vi "BITalino.vi"() -> ()   [LabVIEW 2019]
uses:
  Status.ctl
  Sensor.ctl
  <vilib>/Instr/_visa.llb/VISA Configure Serial Port (Instr).vi
  <vilib>/measure/mamon.llb/Waveform Peak Detection for N Chan.vi
  <vilib>/httpClient/LabVIEWHTTPClient.lvlib
  <vilib>/measure/NI_MAPro.lvlib
panel:
  in  "Tab Control":T1(tab)
  in  "Entrer":bool
  in  "fermer":bool
  in  "reset":bool
  in  "Login":bool
  in  "Pass Word":string
  in  "User Name":string
  in  "Search Button 2":bool
  in  "acquisition 2":bool
  in  "fermer 3":bool
  in  "Home Button":bool
  in  "inscription":bool
  in  "acquisition":bool
  in  "documentation":bool
  in  "Refresh Button2":bool
  in  "Open Button":bool
  in  "Search Button":bool
  in  "fermer 4":bool
  in  "suivant":bool
  in  "sexe":string
  in  "Age":string
  in  "nom":string
  in  "CIN":string
  in  "prenom":string
  in  "Refresh":bool
  in  "envoyer":bool
  out "body":string
  in  "Home Button 2":bool
  out "body 2":string
  in  "CIN":string
  out "body 3":string
  in  "Previous Button":bool
  in  "Jump Button":bool
  in  "Stop Button":bool
  in  "Record Button":bool
  in  "Exit Button":bool
  out "Status":T2
  in  "Device":refnum<visa-resource-name>
  in  "X Limit":u32(knob)=5 scale=2.0..30.0
  in  "File Path":path
  in  "Sample Rate":enum16{"1", "10", "100", "1000"}(ring)=enum."1000"
  in  "MODE":bool
  out "DI 3":bool
  out "DI 4":bool
  out "DI 1":bool
  out "DI 2":bool
  in  "Sensor 1":T3
  in  "Sensor 2":T3=enum."ECG"
  in  "Sensor 3":T3=enum."EEG"
  in  "Sensor 4":T3=enum."EDA"
  in  "Sensor 5":T3=enum."ACC"
  in  "Sensor 6":T3=enum."LUX"
  in  "Sensor Selection":enum32{"A1", "A2", "A3", "A4", "A5", "A6"}(radio)
  out "XY Graph":cluster{dbl[], dbl[]}(graph)
  out "CRC Error":bool
  in  "Battery \nThreshold (%)":u8(slide)=5 min=5 max=90 step=5 scale=5.0..90.0
  in  "DO 1":bool
  in  "DO 2":bool
  in  "DO 3":bool
  in  "DO 4":bool
  in  "Home Button 3":bool
  out "ECG":string[][](table) caption="Table"
  in  "Previous Button 2":bool
  in  "Save Button":bool
  in  "Record Button 2":bool
  out "ecg normal":dbl[](graph)
  in  "Menu Ring":u16(ring) items=["normal", "p interval", "qrs interval", "p-r interval"]
  in  "Home Button 4":bool
  in  "fermer 2":bool
  out "Impulsion":dbl
  out "fréquence en Hz":dbl
  out "Battement de coeur (batt/min)":dbl
  in  "use system alert? (T)":bool=TRUE
  out "Waveform Graph":dynamicdata(graph)
  out "body 4":string
  in  "Jump Button 2":bool
  in  "Previous Button 3":bool
  in  "Home Button 5":bool
  in  "fermer 5":bool
  out "tdms file":refnum<k34>
  out "Ylabel and Plot name":cluster{string, string}
  out "Sample Rate Numeric":i32
  out "Consumer":i32
  out "producer":i32
  in  "error in (no error)":errorcluster
  out "Sync Stop":bool=TRUE
  # "Bienvenue"
  # "Authentification"
  # "Traitement de Signal ECG"
  # "Chercher un Patient"
  # "Formulaire d'inscription"
  # "nom:"
  # "prenom:"
  # "CIN:"
  # "Age:"
  # "Sexe:"
  # "Acquisition de Signal ECG"
  # "LIVE MODE"
  # "SIMULATED MODE"
  # "Hz"
  # "Signal ECG"
  # "Signal ECG"
  # "L'Électrocardiogramme (ECG) est un enregistrement de l'activité électrique du cœur"
  # "Le tracé électrique comporte des ondes et des intervalles entre les ondes :\n\nOnde P : elle correspond à la dépolarisation (et la contraction) des oreillettes. Sa durée (entre 0.08 et 0.1 s) \n\nIntervalle PR (ou PQ) : c'est le temps entre le début de P et le début du \" QRS \". Il est témoins du temps nécessaire à la transmission de l'influx électrique des oreillettes aux ventricules et qui dure 0.12 à 0.20 s.\n\nOnde QRS (appelée aussi complexe QRS) : elle correspond à la dépolarisation (la contraction) des ventricules. une durée de 0.06 à 0.1s.\n\nOnde T : elle correspond à l'essentiel de repolarisation (relaxation des ventricules) et commence juste après QRS et dure de 0.2 à 0.25 s.\n\nIntervalle QT : il est mesuré du débit de QRS à la fin du l'onde T et il correspond à l'ensemble de la repolarisation cardiaque."
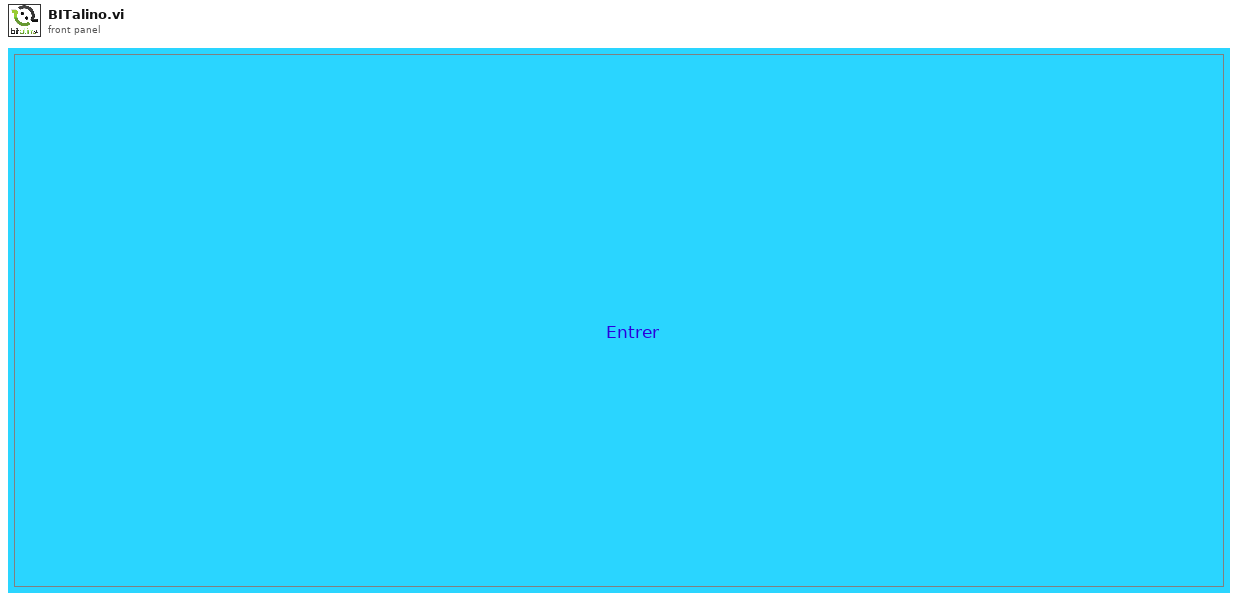
[diagram p1: front panel]
types:
  T1 = enum32{"bienvenue", "Authentification", "acueil", "inscription", "Acquisition", "simulation", "Documentation "}
  T2 = typedef "Status.ctl" = enum16{"Initialize", "Standby", "Recording", "Exit"}
  T3 = typedef "Sensor.ctl" = enum16{"EMG", "ECG", "EEG", "EDA", "ACC", "LUX"}
  T4 = enum8{"Enabled", "Disabled", "Disabled and Grayed Out"}
  T5 = enum16{"open", "open or create", "create or replace", "create", "open (read-only)"}
  T6 = cluster{"Sensor 1":T3, "Sensor 2":T3, "Sensor 3":T3, "Sensor 4":T3, "Sensor 5":T3, "Sensor 6":T3}
  T7 = cluster{"Result":dbl, "Result":dbl, "Result":dbl, "Result":dbl, "Result":dbl, "Result":dbl}
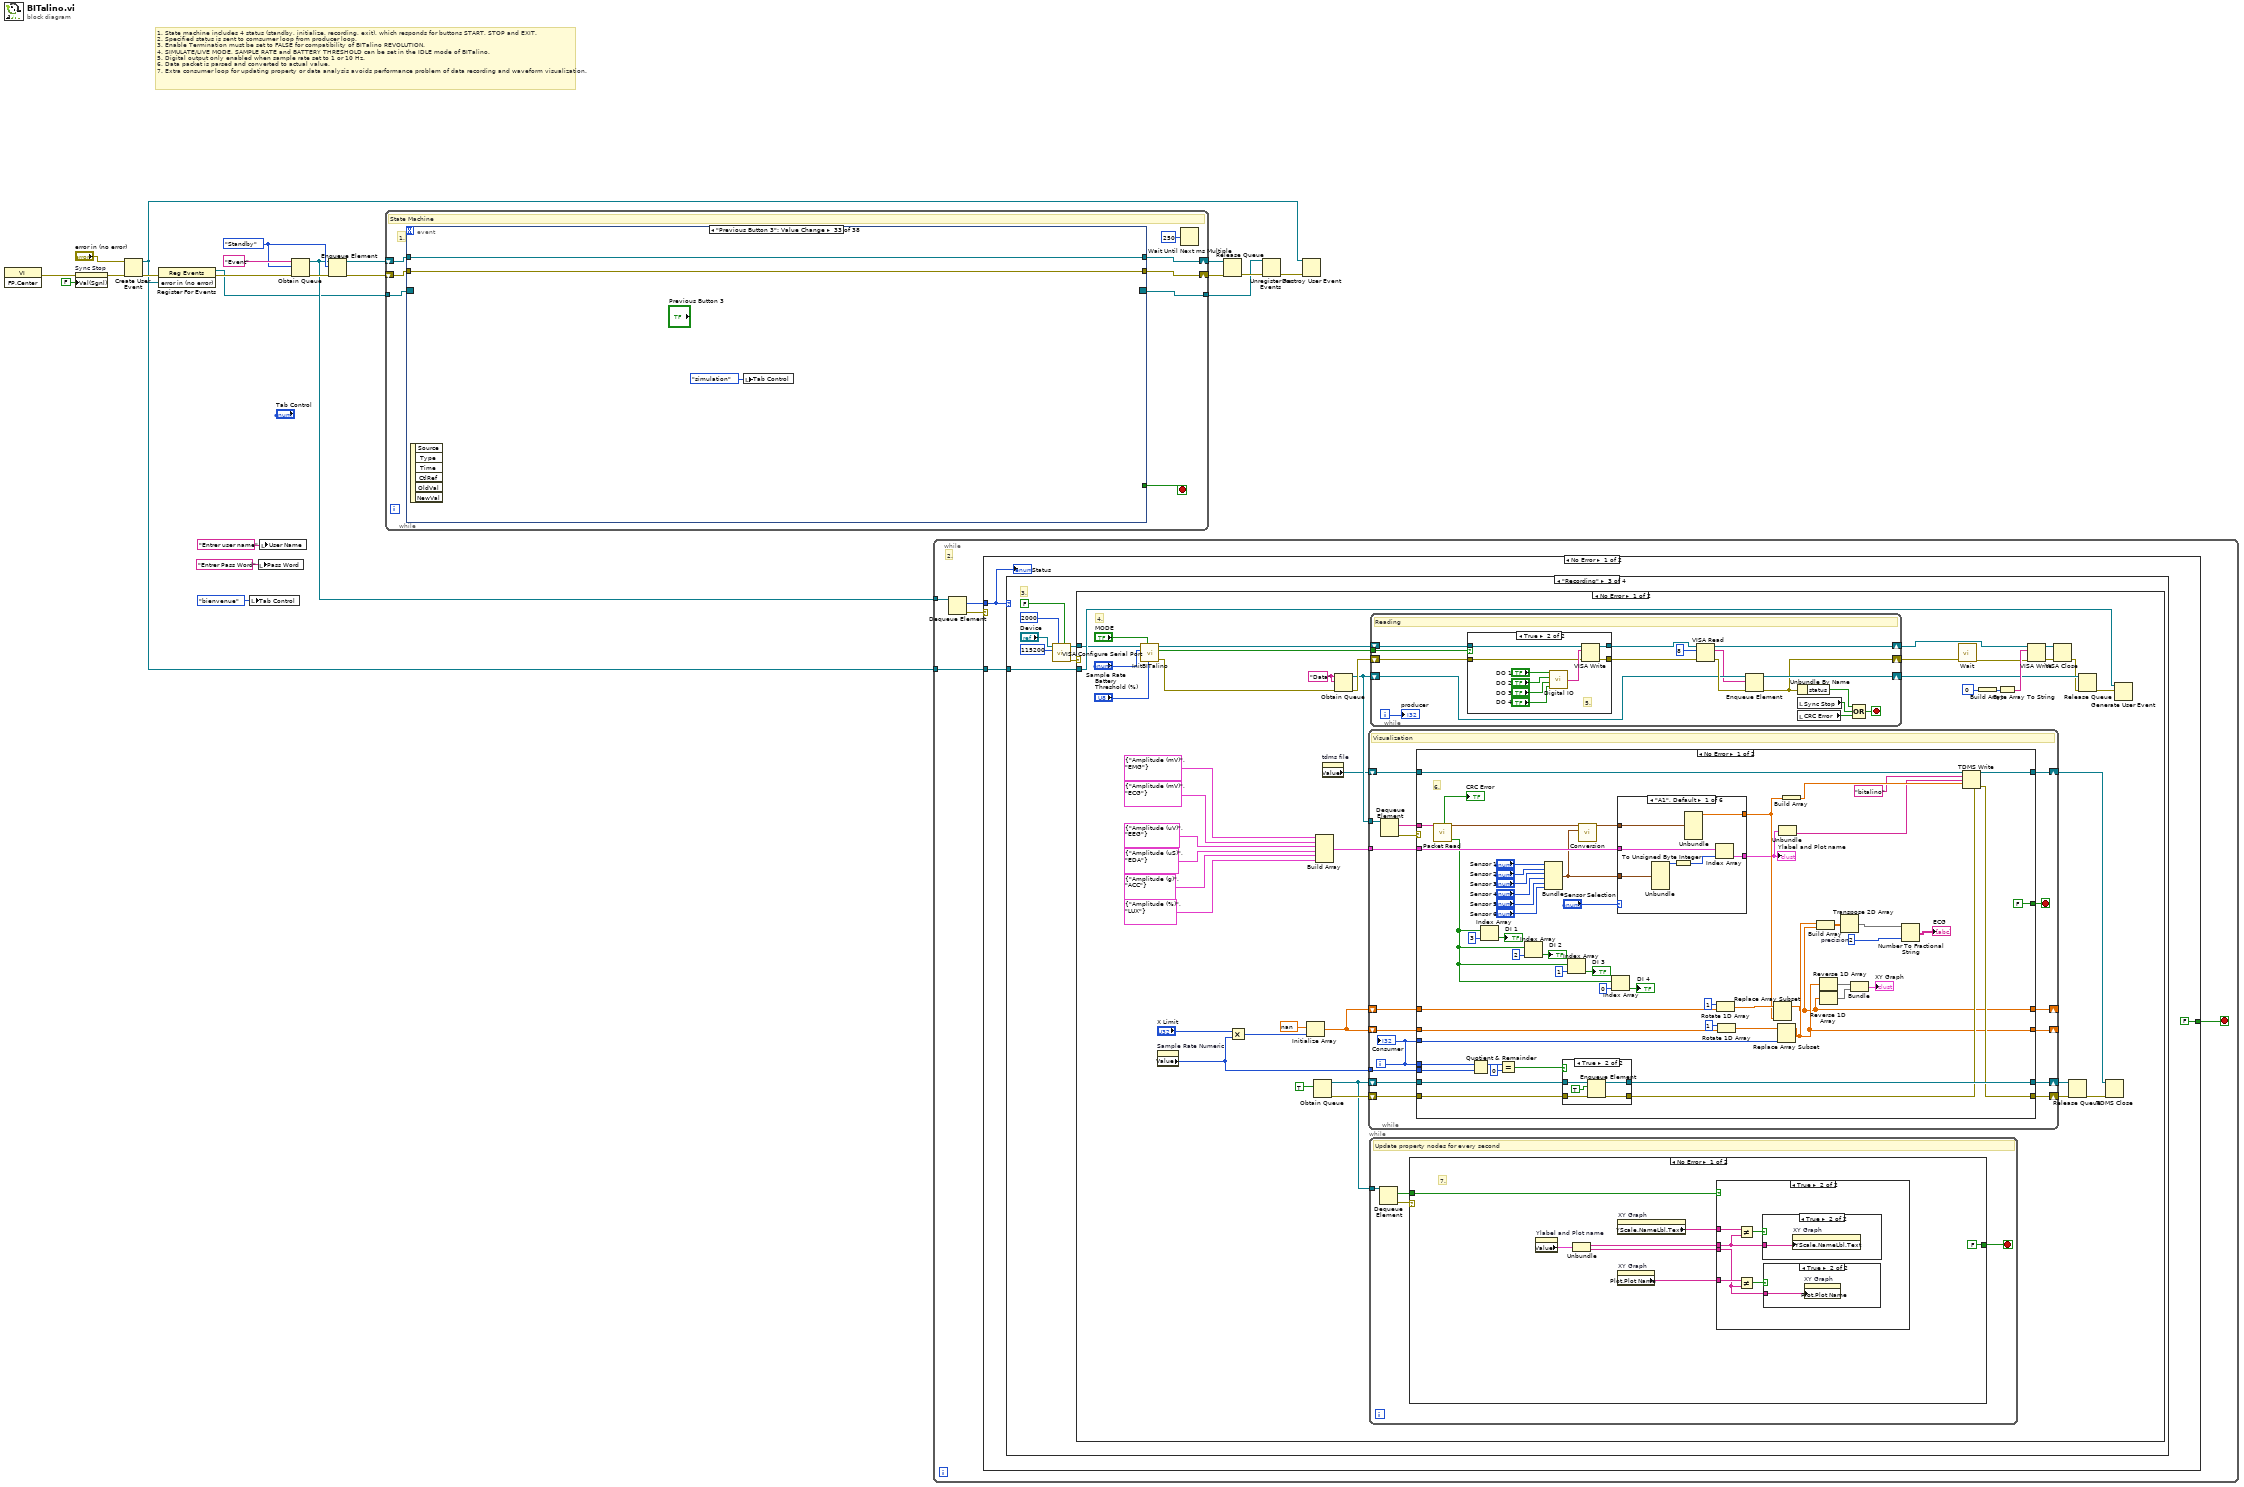
[diagram p0: block diagram]
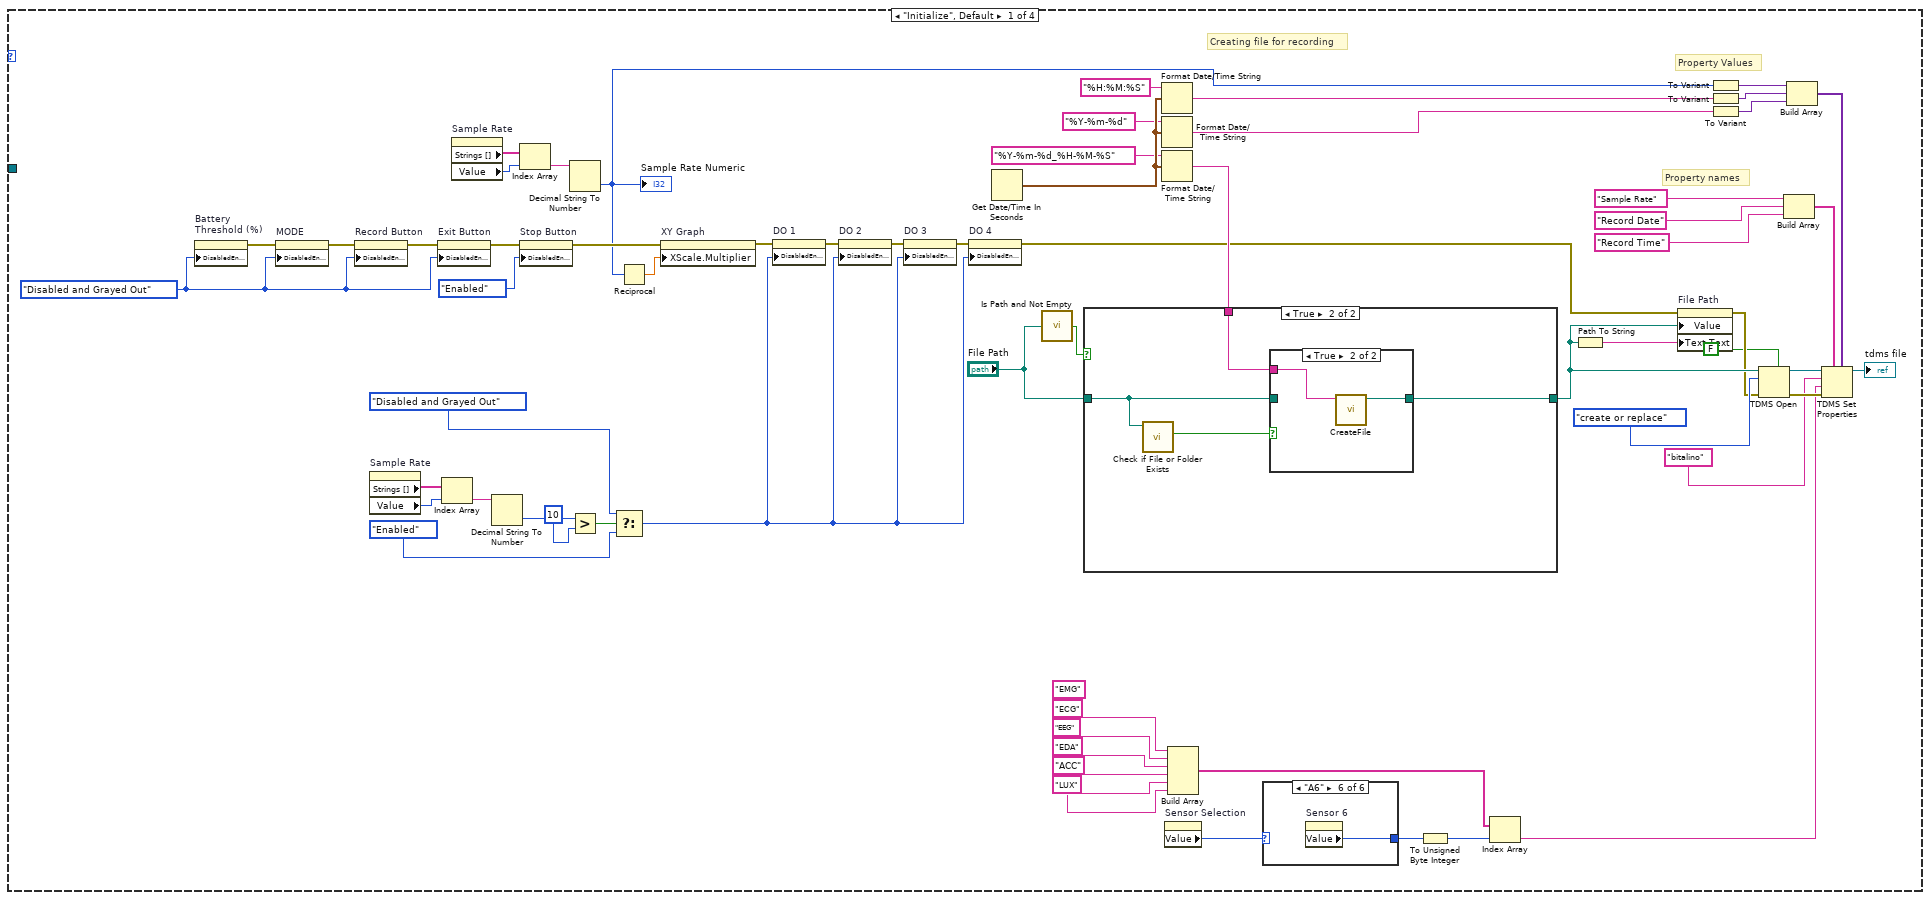
[diagram p2: hidden frame]
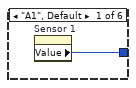
[diagram p3: hidden frame]
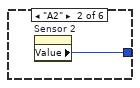
[diagram p4: hidden frame]
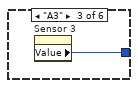
[diagram p5: hidden frame]
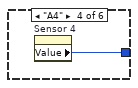
[diagram p6: hidden frame]
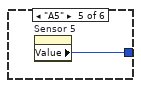
[diagram p7: hidden frame]
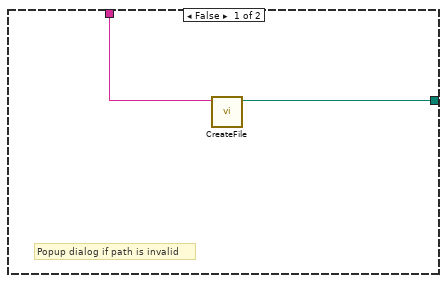
[diagram p8: hidden frame]
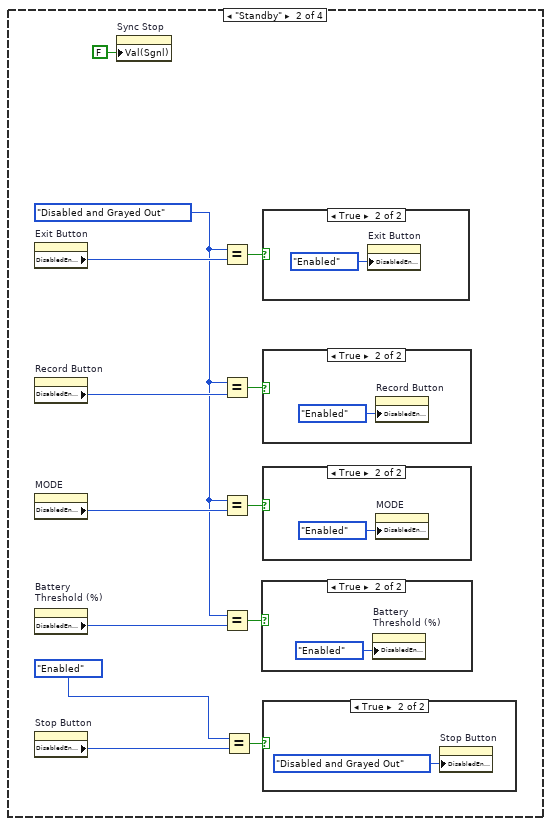
[diagram p10: hidden frame]
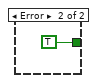
[diagram p19: hidden frame]
diagram:
  w16 = Status."Standby" ("Enum")
  # "1. State machine includes 4 status (standby, initialize, recording, exit), which responds for buttons START, STOP and EXIT.\n2. Specified status is sent to comsumer loop from producer loop.\n3. Enable Termination must be set to FALSE for compatibility of BITalino REVOLUTION.\n4. SIMULATE/LIVE MODE, SAMPLE RATE and BATTERY THRESHOLD can be set in the IDLE mode of BITalino.\n5. Digital output only enabled when sample rate set to 1 or 10 Hz.\n6. Data packet is parsed and converted to actual value.\n7. Extra consumer loop for updating property or data analysis avoids performance problem of data recording and waveform visualization."
  n1 = invoke class="VI" method="FP.Center"() -> (error out=w4:errorcluster)  [unwired: 3 in, 2 out]
  n2 = property on="Sync Stop" class="Bool (strict)"(error in=w4, "Val(Sgnl)"=FALSE ("Value (Signaling)")) -> (error out=w13:errorcluster)  [unwired: 1 in, 1 out]
  n3 = Create User Event(user event datatype="error in (no error)", error in=w13) -> (user event=w5:refnum<user-event>, error out=w12:errorcluster)
  n4 = register-events(error in=w12, w5) -> (reference out=w10:refnum<event-registration>, error out=w11:errorcluster)  [unwired: 1 in]
  n5 = local write "Tab Control"(T1."bienvenue" ("Tab Control")) -> ()
  n6 = local write "Pass Word"("Entrer Pass Word" ("Pass Word")) -> ()
  n7 = local write "User Name"("Entrer user name" ("User Name")) -> ()
  n8 = Obtain Queue(name (unnamed)="Event", element data type=w16, error in (no error)=w11) -> (queue out=w15:refnum<queue>, error out=w19:errorcluster)  [unwired: 2 in, 1 out]
  n9 = Enqueue Element(queue=w15, element=w16, error in (no error)=w19) -> (queue out=w17:refnum<queue>, error out=w18:errorcluster)  [unwired: 1 in, 1 out]
  n10 = while {
    shift-right: [w27] -> w21
    shift-left: w17 -> [w30]
    shift-right: [w28] -> w20
    shift-left: w18 -> [w29]
    tunnel: w10 -> [w24]
    tunnel: [w23] -> w7
    stop <- w26 stop-if-true
    # "1."
    # "State Machine"
    n11 = event shown="[32] \"Previous Button 3\": Value Change" {
      selector: w24 -> [_ _ _ _ _ _ _ _ _ _ _ _ _ _ _ _ _ _ _ _ _ _ _ _ _ _ _ _ _ _ _ _ _ _ _ _ _ _]
      dyn-events: [_ _ _ _ _ _ _ _ _ _ _ _ _ _ _ _ _ _ _ _ _ _ _ _ _ _ _ _ _ _ _ _ _ _ _ _ _ _] -> w23
      timeout: _ -> [_ _ _ _ _ _ _ _ _ _ _ _ _ _ _ _ _ _ _ _ _ _ _ _ _ _ _ _ _ _ _ _ _ _ _ _ _ _]
      tunnel: w30 -> [w37 w40 w57 w60 w63 w66 w69 w72 w75 w78 w84 w86 w89 w92 w104 w107 w109 w113 w128 w135 w144 w147 w172 w186 w194 w197 w200 w203 w206 w210 w213 w216 w219 w223 w227 w231 w241 w245]
      tunnel: w29 -> [w34 w39 w56 w59 w62 w65 w68 w71 w74 w80 w83 w85 w88 w91 w103 w106 w108 w112 w129 w136 w145 w148 w173 w185 w193 w198 w201 w204 w207 w211 w214 w217 w220 w224 w228 w232 w240 w243]
      tunnel: [w31 w39 w56 w59 w62 w65 w68 w71 w74 w81 w83 w85 w88 w91 w103 w106 w108 w112 w129 w136 w145 w148 w173 w185 w193 w198 w201 w204 w207 w211 w214 w217 w220 w224 w228 w232 w235 w242] -> w28
      tunnel: [w38 w40 w57 w60 w63 w66 w69 w72 w75 w79 w84 w86 w89 w92 w104 w107 w109 w113 w128 w135 w144 w147 w172 w186 w194 w197 w200 w203 w206 w210 w213 w216 w219 w223 w227 w231 w237 w244] -> w27
      tunnel: [FALSE _ _ _ _ _ _ _ _ TRUE _ _ _ _ _ _ _ _ _ _ _ _ _ _ _ TRUE _ _ _ TRUE _ _ _ TRUE TRUE TRUE FALSE _] -> w26
      event "Stop Button": Value Change {
        n12 = event-data() -> ()  [unwired: 1 in, 5 out]
        n13 = Enqueue Element(queue=w37, element=Status."Standby" ("Enum"), error in (no error)=w34) -> (queue out=w38:refnum<queue>, error out=w32:errorcluster)  [unwired: 1 in, 1 out]
        n14 = property on="Sync Stop" class="Bool (strict)"(error in=w32, "Val(Sgnl)"=TRUE) -> (error out=w31:errorcluster)  [unwired: 1 in, 1 out]
      }
      event "Menu Ring": Value Change {
        n15 = event-data() -> ()  [unwired: 1 in, 6 out]
        n16 = case shown="1" "Menu Ring" {
          tunnel: [w45 w48 w51 w54] -> w41
          tunnel: ["The condition is NORMAL" "The AV(Atrio Ventricular) Node Blocks - FIRST DEGREE OF HEART ATTACK" "There will be a block in bundle of his - SEVERE HEART ATTACK" "Atrial Depolarisation occurs - HEART ATTACK BEGGINING STAGE "] -> _
          tunnel: [FALSE TRUE TRUE TRUE] -> _
          frame 0, Default {
            w45 = dbl[] [1.0, 1.0, 1.3, 1.0, 1.0, 0.8, 2.5, 0.7, 1.0, 1.0, 1.5, 1.0, 1.0, 1.0]  # normal
          }
          frame 1 {
            w48 = dbl[] [1.0, 1.0, 1.3, 1.0, 1.0, 1.0, 0.8, 2.5, 0.7, 1.0, 1.0, 1.5, 1.0, 1.0, 1.0]  # p-r interval
            # "p-r interval"
          }
          frame 2 {
            w51 = dbl[] [1.0, 1.0, 1.3, 1.0, 1.0, 0.8, 1.65, 2.5, 1.6, 0.7, 1.0, 1.0, 1.5, 1.0, 1.0, 1.0]  # qrs interval
            # "qrs interval"
          }
          frame 3 {
            w54 = dbl[] [1.0, 1.0, 1.1, 1.3, 1.1, 1.0, 0.8, 2.5, 0.7, 1.0, 1.0, 1.5, 1.0, 1.0, 1.0]  # p interval
            # "p interval"
          }
        }
        "ecg normal" <- w41
      }
      event "Jump Button": Value Change {
        n17 = event-data() -> ()  [unwired: 1 in, 6 out]
        n18 = local write "Tab Control"(T1."Documentation " ("Tab Control")) -> ()
      }
      event "documentation": Value Change {
        n19 = event-data() -> ()  [unwired: 1 in, 6 out]
        n20 = local write "Tab Control"(T1."Documentation " ("Tab Control")) -> ()
      }
      event "Home Button": Value Change {
        n21 = event-data() -> ()  [unwired: 1 in, 6 out]
        n22 = local write "Tab Control"(T1."acueil" ("Tab Control")) -> ()
      }
      event "Home Button 2": Value Change {
        n23 = event-data() -> ()  [unwired: 1 in, 6 out]
        n24 = local write "Tab Control"(T1."acueil" ("Tab Control")) -> ()
      }
      event "Home Button 3": Value Change {
        n25 = event-data() -> ()  [unwired: 1 in, 6 out]
        n26 = local write "Tab Control"(T1."acueil" ("Tab Control")) -> ()
      }
      event "Home Button 4": Value Change {
        n27 = event-data() -> ()  [unwired: 1 in, 6 out]
        n28 = local write "Tab Control"(T1."acueil" ("Tab Control")) -> ()
      }
      event "Previous Button": Value Change {
        n29 = event-data() -> ()  [unwired: 1 in, 6 out]
        n30 = local write "Tab Control"(T1."inscription" ("Tab Control")) -> ()
      }
      event "Exit Button": Value Change {
        n31 = event-data() -> ()  [unwired: 1 in, 5 out]
        n32 = Enqueue Element(queue=w78, element=Status."Exit" ("Enum"), error in (no error)=w80) -> (queue out=w79:refnum<queue>, error out=w81:errorcluster)  [unwired: 1 in, 1 out]
      }
      event "Entrer": Value Change {
        n33 = event-data() -> ()  [unwired: 1 in, 5 out]
        n34 = local write "Tab Control"(T1."Authentification" ("Tab Control")) -> ()
      }
      event "User Name": Mouse Down {
        n35 = event-data() -> ()  [unwired: 1 in, 5 out]
        n36 = local write "User Name"("" ("User Name")) -> ()
      }
      event "Pass Word": Mouse Down {
        n37 = event-data() -> ()  [unwired: 1 in, 5 out]
        n38 = local write "Pass Word"("" ("Pass Word")) -> ()
      }
      event "Login": Value Change {
        n39 = event-data() -> ()  [unwired: 1 in, 5 out]
        n40 = Equal?(x="Pass Word", y="12345") -> (x = y?=w94:bool)
        n41 = Equal?(x="User Name", y="Imen") -> (x = y?=w95:bool)
        n42 = And(x=w95, y=w94) -> (x .and. y?=w93:bool)
        n43 = case shown="True" w93 {
          frame False {
            n44 = call "Display Message to User"("Enable"=TRUE) -> ()  [unwired: 9 in, 2 out]
          }
          frame True {
            n45 = local write "Tab Control"(T1."acueil" ("Tab Control")) -> ()
          }
        }
      }
      event "inscription": Value Change {
        n46 = event-data() -> ()  [unwired: 1 in, 6 out]
        n47 = local write "Tab Control"(T1."inscription" ("Tab Control")) -> ()
      }
      event "acquisition": Value Change {
        n48 = event-data() -> ()  [unwired: 1 in, 6 out]
        n49 = local write "Tab Control"(T1."Acquisition" ("Tab Control")) -> ()
      }
      event "reset": Value Change {
        n50 = event-data() -> ()  [unwired: 1 in, 6 out]
        n51 = local write "Pass Word"("" ("Pass Word")) -> ()
        n52 = local write "User Name"("" ("User Name")) -> ()
      }
      event "envoyer": Value Change {
        n53 = event-data() -> ()  [unwired: 1 in, 6 out]
        n54 = case shown="True" "envoyer" {
          frame False {
          }
          frame True {
            n55 = Concatenate Strings("localhost/fiche.php?n=" ("string"), "nom", "&p=" ("string"), "prenom", "&c=" ("string"), "CIN", "&a=" ("string"), "Age", "&s=" ("string"), "sexe") -> (w116:string)
            n56 = call <vilib>:"GET.vi"("url"=w116) -> ("body"=→"body":string)  [unwired: 11 in, 3 out]
          }
        }
      }
      event "Search Button": Value Change {
        n57 = event-data() -> ()  [unwired: 1 in, 6 out]
        n58 = case shown="True" "Search Button" {
          frame False {
          }
          frame True {
            n59 = Concatenate Strings("localhost/chercherpatient.php?cin=" ("string"), "CIN") -> (w131:string)
            n60 = call <vilib>:"GET.vi"("url"=w131) -> ("body"=→"body 2":string)  [unwired: 11 in, 3 out]
          }
        }
      }
      event "Open Button": Value Change {
        n61 = event-data() -> ()  [unwired: 1 in, 6 out]
        n62 = case shown="True" "Open Button" {
          frame False {
          }
          frame True {
            n63 = local read "CIN"() -> (w137:string)
            n64 = Concatenate Strings("localhost/details.php?cin=" ("string"), w137) -> (w139:string)
            n65 = call <vilib>:"GET.vi"("url"=w139) -> ("body"=→"body 3":string)  [unwired: 11 in, 3 out]
          }
        }
      }
      event "Refresh Button2": Value Change {
        n66 = event-data() -> ()  [unwired: 1 in, 6 out]
        n67 = local write "CIN"("" ("cin")) -> ()
        n68 = local write "body 2"("" ("body 2")) -> ()
        n69 = local write "body 3"("" ("body 3")) -> ()
      }
      event "Record Button 2": Value Change {
        n70 = event-data() -> ()  [unwired: 1 in, 6 out]
        n71 = for {
          N: 130 -> [_]
          n72 = call "Simulate Signal"() -> ("Sawtooth with Uniform Noise"=w155:dynamicdata)  [unwired: 14 in, 1 out]
          n73 = call "Filter"("Signal"=w155) -> ("Filtered Signal"=w167:dynamicdata)  [unwired: 9 in, 1 out]
          n74 = call "Filter2"("Signal"=w167) -> ("Filtered Signal"=w166:dynamicdata)  [unwired: 9 in, 1 out]
          n75 = call "Collector"("Signals"=w166) -> ("Collected Signals"=w151:dynamicdata)  [unwired: 9 in, 1 out]
          "Waveform Graph" <- w151
          n76 = call "Statistics"("Signals"=w151) -> ("Maximum"=w154:dynamicdata)  [unwired: 25 in, 1 out]
          n77 = call "Convert from Dynamic Data"("Dynamic Data Type"=w154) -> ("Scalar"=w164:dbl)  [unwired: 3 in]
          n78 = Multiply(x=w164, y=0.6) -> (x*y=w163:dbl)
          n79 = call-poly <vilib>:"Waveform Peak Detection.vi"("width"=15, "threshold"=w163, "Signals In"=w151) -> ("# found"=w161:i32[])  [unwired: 4 in, 4 out]
          n80 = call "Convert to Dynamic Data"("Array"=w161) -> ("Dynamic Data Type"=w150:dynamicdata)  [unwired: 3 in]
          n81 = Wait Until Next ms Multiple(millisecond multiple=u32 100) -> ()  [unwired: 1 out]
          n82 = call "Convert from Dynamic Data2"("Dynamic Data Type"=w150) -> ("Scalar"=w160:dbl)  [unwired: 3 in]
          "Impulsion" <- w160
          n83 = Greater?(x=w150, y=15.0) -> (0:w153:dynamicdata)
          n84 = case shown="True" w153 {
            frame False {
            }
            frame True {
              n85 = call <vilib>:"Beep.vi"("use system alert? (T)"="use system alert? (T)", "duration (msec)"=u32 500, "frequency (Hz)"=u32 4000) -> ()  [unwired: 9 in]
            }
          }
          n86 = Divide(x=w160, y=15.0) -> (x/y=w157:dbl)
          "fréquence en Hz" <- w157
          n87 = Multiply(x=w157, y=60.0) -> (x*y=→"Battement de coeur (batt/min)":dbl)
        }
      }
      event "Save Button": Value Change {
        n88 = event-data() -> ()  [unwired: 1 in, 6 out]
        n89 = case shown="True" "Save Button" {
          frame False {
          }
          frame True {
            n90 = local read "Battement de coeur (batt/min)"() -> (w176:dbl)
            n91 = local read "fréquence en Hz"() -> (w180:dbl)
            n92 = local read "Impulsion"() -> (w183:dbl)
            n93 = Format Into String(w183) -> (resulting string=w182:string)  [unwired: 3 in, 1 out]
            n94 = Format Into String(w180) -> (resulting string=w179:string)  [unwired: 3 in, 1 out]
            n95 = Format Into String(w176) -> (resulting string=w177:string)  [unwired: 3 in, 1 out]
            n96 = Concatenate Strings("localhost/ecg.php?i=" ("string"), w182, "&f=" ("string"), w179, "&b=" ("string"), w177) -> (w175:string)
            n97 = call <vilib>:"GET.vi"("url"=w175) -> ("body"=→"body 4":string)  [unwired: 11 in, 3 out]
          }
        }
      }
      event "Refresh": Value Change {
        n98 = event-data() -> ()  [unwired: 1 in, 6 out]
        n99 = local write "prenom"("" ("prenom")) -> ()
        n100 = local write "nom"("" ("nom")) -> ()
        n101 = local write "CIN"("" ("CIN")) -> ()
        n102 = local write "Age"("" ("Age")) -> ()
        n103 = local write "sexe"("" ("sexe")) -> ()
      }
      event "suivant": Value Change {
        n104 = event-data() -> ()  [unwired: 1 in, 6 out]
        n105 = local write "Tab Control"(T1."Acquisition" ("Tab Control")) -> ()
      }
      event "fermer": Value Change {
        n106 = event-data() -> ()  [unwired: 1 in, 6 out]
        n107 = local write "Tab Control"(T1."bienvenue" ("Tab Control")) -> ()
      }
      event "acquisition 2": Value Change {
        n108 = event-data() -> ()  [unwired: 1 in, 6 out]
        n109 = local write "Tab Control"(T1."simulation" ("Tab Control")) -> ()
      }
      event "Search Button 2": Value Change {
        n110 = event-data() -> ()  [unwired: 1 in, 6 out]
        n111 = local write "Tab Control"(T1."inscription" ("Tab Control")) -> ()
      }
      event "Home Button 5": Value Change {
        n112 = event-data() -> ()  [unwired: 1 in, 6 out]
        n113 = local write "Tab Control"(T1."acueil" ("Tab Control")) -> ()
      }
      event "fermer 5": Value Change {
        n114 = event-data() -> ()  [unwired: 1 in, 6 out]
        n115 = local write "Tab Control"(T1."bienvenue" ("Tab Control")) -> ()
      }
      event "Jump Button 2": Value Change {
        n116 = event-data() -> ()  [unwired: 1 in, 6 out]
        n117 = local write "Tab Control"(T1."Documentation " ("Tab Control")) -> ()
      }
      event "Previous Button 2": Value Change {
        n118 = event-data() -> ()  [unwired: 1 in, 6 out]
        n119 = local write "Tab Control"(T1."Acquisition" ("Tab Control")) -> ()
      }
      event "Previous Button 3": Value Change {
        n120 = event-data() -> ()  [unwired: 1 in, 6 out]
        n121 = local write "Tab Control"(T1."simulation" ("Tab Control")) -> ()
      }
      event "fermer 2": Value Change {
        n122 = event-data() -> ()  [unwired: 1 in, 6 out]
        n123 = local write "Tab Control"(T1."bienvenue" ("Tab Control")) -> ()
      }
      event "fermer 3": Value Change {
        n124 = event-data() -> ()  [unwired: 1 in, 6 out]
        n125 = local write "Tab Control"(T1."bienvenue" ("Tab Control")) -> ()
      }
      event "fermer 4": Value Change {
        n126 = event-data() -> ()  [unwired: 1 in, 6 out]
        n127 = local write "Tab Control"(T1."bienvenue" ("Tab Control")) -> ()
      }
      event "Record Button": Value Change {
        n128 = event-data() -> ()  [unwired: 1 in, 1 out]
        n129 = Enqueue Element(queue=w241, element=Status."Initialize" ("Enum"), error in (no error)=w240) -> (queue out=w238:refnum<queue>, error out=w236:errorcluster)  [unwired: 1 in, 1 out]
        n130 = Enqueue Element(queue=w238, element=Status."Recording" ("Enum"), error in (no error)=w236) -> (queue out=w237:refnum<queue>, error out=w235:errorcluster)  [unwired: 1 in, 1 out]
      }
      event User Event {
        n131 = event-data() -> ()  [unwired: 1 in, 1 out]
        n132 = Enqueue Element(queue=w245, element=Status."Standby" ("Enum"), error in (no error)=w243) -> (queue out=w244:refnum<queue>, error out=w242:errorcluster)  [unwired: 1 in, 1 out]
      }
    }
    n133 = Wait Until Next ms Multiple(millisecond multiple=u32 250) -> ()  [unwired: 1 out]
  }
  n134 = while {
    tunnel: w15 -> [w250]
    tunnel: w5 -> [w247]
    stop <- w251 stop-if-true
    # "2."
    n135 = Dequeue Element(queue=w250) -> (element=w249:T2, error out=w248:errorcluster)  [unwired: 2 in, 2 out]
    n136 = case shown="No Error" w248 {
      tunnel: w249 -> [w253 _]
      tunnel: [FALSE TRUE] -> w251
      tunnel: w247 -> [w252 _]
      frame No Error {
        n137 = case shown="\"Recording\"" w253 {
          tunnel: w252 -> [_ _ w351 _]
          frame "Initialize", Default {
            w282 = T4."Disabled and Grayed Out" ("Disabled")
            # "Creating file for recording"
            # "Property Values"
            # "Property names"
            n138 = property on="Battery \nThreshold (%)" class="Slide (strict)"("DisabledEnum"=w282) -> (error out=w283:errorcluster)  [unwired: 2 in, 1 out]
            n139 = property on="MODE" class="Bool (strict)"(error in=w283, "DisabledEnum"=w282) -> (error out=w309:errorcluster)  [unwired: 1 in, 1 out]
            n140 = property on="Record Button" class="Bool"(error in=w309, "DisabledEnum"=w282) -> (error out=w317:errorcluster)  [unwired: 1 in, 1 out]
            n141 = property on="Sample Rate" class="Enum (strict)"() -> ("Strings []"=w272:string[], "Value"=w271:enum16{"1", "10", "100", "1000"})  [unwired: 2 in, 2 out]
            n142 = property on="Exit Button" class="Bool"(error in=w317, "DisabledEnum"=w282) -> (error out=w315:errorcluster)  [unwired: 1 in, 1 out]
            n143 = Index Array(array=w272, index=w271) -> (element=w270:string)
            n144 = property on="Sample Rate" class="Enum (strict)"() -> ("Strings []"=w314:string[], "Value"=w313:enum16{"1", "10", "100", "1000"})  [unwired: 2 in, 2 out]
            n145 = Decimal String To Number(string=w270) -> (number=w269:i32)  [unwired: 2 in, 1 out]
            n146 = Index Array(array=w314, index=w313) -> (element=w312:string)
            n147 = property on="Stop Button" class="Bool"(error in=w315, "DisabledEnum"=T4."Enabled" ("Disabled")) -> (error out=w311:errorcluster)  [unwired: 1 in, 1 out]
            n148 = Decimal String To Number(string=w312) -> (number=w281:i32)  [unwired: 2 in, 1 out]
            "Sample Rate Numeric" <- w281
            n149 = Greater?(x=w269, y=10) -> (0:w277:bool)
            n150 = Select(t=T4."Disabled and Grayed Out" ("Disabled"), s=w277, f=T4."Enabled" ("Disabled")) -> (s? t:f=w280:T4)
            n151 = Reciprocal(x=w281) -> (1/x=w310:dbl)
            n152 = property on="XY Graph" class="XYGraph (strict)"(error in=w311, "XScale.Multiplier"=w310) -> (error out=w268:errorcluster)  [unwired: 1 in, 1 out]
            n153 = property on="DO 1" class="Bool (strict)"(error in=w268, "DisabledEnum"=w280) -> (error out=w275:errorcluster)  [unwired: 1 in, 1 out]
            n154 = property on="DO 2" class="Bool (strict)"(error in=w275, "DisabledEnum"=w280) -> (error out=w274:errorcluster)  [unwired: 1 in, 1 out]
            n155 = property on="DO 3" class="Bool (strict)"(error in=w274, "DisabledEnum"=w280) -> (error out=w273:errorcluster)  [unwired: 1 in, 1 out]
            n156 = property on="DO 4" class="Bool (strict)"(error in=w273, "DisabledEnum"=w280) -> (error out=w267:errorcluster)  [unwired: 1 in, 1 out]
            n157 = Get Date/Time In Seconds() -> (seconds since 1Jan1904=w299:timestamp)
            n158 = call <vilib>:"Is Path and Not Empty.vi"("path"="File Path") -> ("Is Path and Not Empty?"=w291:bool)  [unwired: 4 in]
            n159 = Format Date/Time String(time format string (%c)="%H:%M:%S", seconds (now)=w299) -> (date/time string=w304:string)  [unwired: 1 in]
            n160 = Format Date/Time String(time format string (%c)="%Y-%m-%d", seconds (now)=w299) -> (date/time string=w305:string)  [unwired: 1 in]
            n161 = Format Date/Time String(time format string (%c)="%Y-%m-%d_%H-%M-%S", seconds (now)=w299) -> (date/time string=w295:string)  [unwired: 1 in]
            n162 = case shown="True" w291 {
              tunnel: [w324 w327] -> w288
              tunnel: "File Path" -> [_ w326]
              tunnel: w295 -> [w325 w328]
              frame False {
                # "Popup dialog if path is invalid"
                n163 = call "CreateFile.vi"("date/time string"=w325) -> ("appended path"=w324:path)  [unwired: 10 in]
              }
              frame True {
                n164 = call <vilib>:"Check if File or Folder Exists.vi"("path"=w326) -> ("file or folder exists?"=w329:bool)  [unwired: 8 in, 2 out]
                n165 = case shown="True" w329 {
                  tunnel: w328 -> [_ w332]
                  tunnel: [w330 w331] -> w327
                  tunnel: w326 -> [w330 _]
                  frame False {
                  }
                  frame True {
                    n166 = call "CreateFile.vi"("date/time string"=w332) -> ("appended path"=w331:path)  [unwired: 10 in]
                  }
                }
              }
            }
            n167 = property on="Sensor Selection" class="RadioBtnsControl (strict)"() -> ("Value"=w265:enum32{"A1", "A2", "A3", "A4", "A5", "A6"})  [unwired: 2 in, 2 out]
            n168 = Build Array("EMG", "ECG", "EEG", "EDA", "ACC", "LUX") -> (w256:string[])
            n169 = case shown="\"A6\"" w265 {
              tunnel: [w318 w319 w320 w321 w322 w323] -> w258
              frame "A1", Default {
                n170 = property on="Sensor 1" class="Enum (strict)"() -> ("Value"=w318:T3)  [unwired: 2 in, 2 out]
              }
              frame "A2" {
                n171 = property on="Sensor 2" class="Enum (strict)"() -> ("Value"=w319:T3)  [unwired: 2 in, 2 out]
              }
              frame "A3" {
                n172 = property on="Sensor 3" class="Enum (strict)"() -> ("Value"=w320:T3)  [unwired: 2 in, 2 out]
              }
              frame "A4" {
                n173 = property on="Sensor 4" class="Enum (strict)"() -> ("Value"=w321:T3)  [unwired: 2 in, 2 out]
              }
              frame "A5" {
                n174 = property on="Sensor 5" class="Enum (strict)"() -> ("Value"=w322:T3)  [unwired: 2 in, 2 out]
              }
              frame "A6" {
                n175 = property on="Sensor 6" class="Enum (strict)"() -> ("Value"=w323:T3)  [unwired: 2 in, 2 out]
              }
            }
            n176 = To Unsigned Byte Integer(number=w258) -> (unsigned 8bit integer=w257:u8)
            n177 = Index Array(array=w256, index=w257) -> (element=w255:string)
            n178 = Path To String(path=w288) -> (string=w289:string)
            n179 = property on="File Path" class="Path"(error in=w267, "Value"=w288, "Text.Text"=w289) -> (error out=w286:errorcluster)  [unwired: 1 in, 1 out]
            n180 = To Variant(anything=w281) -> (Variant=w303:variant)
            n181 = To Variant(anything=w304) -> (Variant=w306:variant)
            n182 = To Variant(anything=w305) -> (Variant=w307:variant)
            n183 = TDMS Open(5:FALSE ("create index file? (T)"), 8:w286, 10:T5."create or replace" ("operation (0:open)"), 11:w288) -> (0:w294:errorcluster, 3:w293:refnum<k34>)  [unwired: 3 in]
            n184 = Build Array("Sample Rate", "Record Date", "Record Time") -> (w302:string[])
            n185 = Build Array(w303, w306, w307) -> (w308:variant[])
            n186 = TDMS Set Properties(5:w308, 7:w302, 8:w294, 9:w255, 10:"bitalino", 11:w293) -> (3:→"tdms file":refnum<k34>)  [unwired: 3 out]
          }
          frame "Standby" {
            w333 = T4."Disabled and Grayed Out" ("Disabled")
            n187 = property on="Exit Button" class="Bool"() -> ("DisabledEnum"=w344:T4)  [unwired: 2 in, 2 out]
            n188 = property on="Record Button" class="Bool"() -> ("DisabledEnum"=w342:T4)  [unwired: 2 in, 2 out]
            n189 = property on="MODE" class="Bool (strict)"() -> ("DisabledEnum"=w336:T4)  [unwired: 2 in, 2 out]
            n190 = property on="Battery \nThreshold (%)" class="Slide (strict)"() -> ("DisabledEnum"=w334:T4)  [unwired: 2 in, 2 out]
            n191 = property on="Stop Button" class="Bool"() -> ("DisabledEnum"=w339:T4)  [unwired: 2 in, 2 out]
            n192 = property on="Sync Stop" class="Bool (strict)"("Val(Sgnl)"=FALSE ("Value (Signaling)")) -> ()  [unwired: 2 in, 2 out]
            n193 = Equal?(x=w333, y=w344) -> (x = y?=w343:bool)
            n194 = Equal?(x=w333, y=w342) -> (x = y?=w341:bool)
            n195 = Equal?(x=w333, y=w336) -> (x = y?=w337:bool)
            n196 = Equal?(x=w333, y=w334) -> (x = y?=w335:bool)
            n197 = Equal?(x=T4."Enabled" ("Disabled"), y=w339) -> (x = y?=w338:bool)
            n198 = case shown="True" w335 {
              frame False {
              }
              frame True {
                n199 = property on="Battery \nThreshold (%)" class="Slide (strict)"("DisabledEnum"=T4."Enabled" ("Disabled")) -> ()  [unwired: 2 in, 2 out]
              }
            }
            n200 = case shown="True" w343 {
              frame False {
              }
              frame True {
                n201 = property on="Exit Button" class="Bool"("DisabledEnum"=T4."Enabled" ("Disabled")) -> ()  [unwired: 2 in, 2 out]
              }
            }
            n202 = case shown="True" w341 {
              frame False {
              }
              frame True {
                n203 = property on="Record Button" class="Bool"("DisabledEnum"=T4."Enabled" ("Disabled")) -> ()  [unwired: 2 in, 2 out]
              }
            }
            n204 = case shown="True" w337 {
              frame False {
              }
              frame True {
                n205 = property on="MODE" class="Bool (strict)"("DisabledEnum"=T4."Enabled" ("Disabled")) -> ()  [unwired: 2 in, 2 out]
              }
            }
            n206 = case shown="True" w338 {
              frame False {
              }
              frame True {
                n207 = property on="Stop Button" class="Bool"("DisabledEnum"=T4."Disabled and Grayed Out" ("Disabled")) -> ()  [unwired: 2 in, 2 out]
              }
            }
          }
          frame "Recording" {
            # "3."
            n208 = call-poly "VISA Configure Serial Port"("VISA resource name"="Device", "timeout (10sec)"=u32 2000, "Enable Termination\nChar (T)"=FALSE ("Enable Termination\nChar (T)"), "baud rate (9600)"=u32 115200) -> ("VISA resource name out"=w354:refnum<visa-resource-name>, "error out"=w353:errorcluster)  [unwired: 10 in]
            n209 = case shown="No Error" w353 {
              selector: w353 -> [_ w576]
              tunnel: w354 -> [w384 _]
              tunnel: w351 -> [w386 w577]
              frame No Error {
                w394 = "Data"
                # "4."
                n210 = call "InitBITalino.vi"("Battery \nThreshold (%)"="Battery \nThreshold (%)", "MODE"="MODE", "Sample Rate"="Sample Rate", "BITalino"=w384) -> ("error out"=w358:errorcluster, "Digital Output"=w359:bool, "VISA out"=w361:refnum<visa-resource-name>)  [unwired: 5 in]
                n211 = property on="Sample Rate Numeric" class="DigNum (strict)"() -> ("Value"=w375:i32)  [unwired: 2 in, 2 out]
                n212 = Multiply(x="X Limit", y=w375) -> (x*y=w373:u32)
                n213 = Initialize Array(nan ("element"), w373) -> (w372:dbl[])
                n214 = Obtain Queue(element data type=TRUE) -> (queue out=w378:refnum<queue>, error out=w380:errorcluster)  [unwired: 4 in, 1 out]
                n215 = Build Array(cluster{string, string} {"Amplitude (mV)", "EMG"}, cluster{string, string} {"Amplitude (mV)", "ECG"}, cluster{string, string} {"Amplitude (uV)", "EEG"}, cluster{string, string} {"Amplitude (uS)", "EDA"}, cluster{string, string} {"Amplitude (g)", "ACC"}, cluster{string, string} {"Amplitude (%)", "LUX"}) -> (w365:cluster{string, string}[])
                n216 = property on="tdms file" class="Ref (strict)"() -> ("Value"=w364:refnum<k34>)  [unwired: 2 in, 2 out]
                n217 = Obtain Queue(name (unnamed)=w394, element data type=w394, error in (no error)=w358) -> (queue out=w395:refnum<queue>, error out=w396:errorcluster)  [unwired: 2 in, 1 out]
                n218 = while {
                  tunnel: w395 -> [w436]
                  shift-right: [w431] -> _
                  shift-left: w372 -> [w432]
                  tunnel: w375 -> [w430]
                  shift-right: [w427] -> w377
                  shift-left: w378 -> [w429]
                  shift-right: [w426] -> w376
                  shift-left: w380 -> [w428]
                  shift-right: [w423] -> _
                  shift-left: w372 -> [w425]
                  tunnel: w365 -> [w422]
                  shift-right: [w420] -> w362
                  shift-left: w364 -> [w421]
                  i -> [w424]
                  stop <- w434 stop-if-true
                  # "Visualization"
                  n219 = Dequeue Element(queue=w436) -> (element=w433:string, error out=w435:errorcluster)  [unwired: 2 in, 2 out]
                  n220 = case shown="No Error" w435 {
                    tunnel: [FALSE TRUE] -> w434
                    tunnel: w433 -> [w458 _]
                    tunnel: w432 -> [w476 w546]
                    tunnel: [w438 w546] -> w431
                    tunnel: w430 -> [w477 _]
                    tunnel: w424 -> [w482 _]
                    tunnel: w429 -> [w485 w545]
                    tunnel: w428 -> [w484 w544]
                    tunnel: [w483 w545] -> w427
                    tunnel: [w460 w544] -> w426
                    tunnel: w425 -> [w473 w543]
                    tunnel: w424 -> [w470 _]
                    tunnel: [w439 w543] -> w423
                    tunnel: w422 -> [w469 _]
                    tunnel: w421 -> [w465 w542]
                    tunnel: [w464 w542] -> w420
                    frame No Error {
                      w443 = 2  # precision
                      # "6."
                      n221 = call "Packet Read.vi"("Packets"=w458) -> ("Digital IO"=w449:bool[], "Analog Channels"=w457:cluster{u16, u16, u16, u16, u16, u16}, "CRC Error"=→"CRC Error":bool)  [unwired: 7 in, 1 out]
                      n222 = Quotient & Remainder(x=w482, y=w477) -> (x-y*floor(x/y)=w481:i32)  [unwired: 1 out]
                      n223 = Index Array(array=w449, index=3) -> (element=→"DI 1":bool)
                      n224 = Equal?(x=w481, y=0) -> (x = y?=w479:bool)
                      n225 = Index Array(array=w449, index=2) -> (element=→"DI 2":bool)
                      n226 = Bundle("Sensor 1"="Sensor 1", "Sensor 2"="Sensor 2", "Sensor 3"="Sensor 3", "Sensor 4"="Sensor 4", "Sensor 5"="Sensor 5", "Sensor 6"="Sensor 6") -> (w468:T6)  [unwired: 1 in]
                      n227 = case shown="True" w479 {
                        tunnel: w485 -> [w494 w499]
                        tunnel: w484 -> [w493 w498]
                        tunnel: [w494 w497] -> w483
                        tunnel: [w493 w496] -> w463
                        frame False {
                        }
                        frame True {
                          n228 = Enqueue Element(queue=w499, element=TRUE, error in (no error)=w498) -> (queue out=w497:refnum<queue>, error out=w496:errorcluster)  [unwired: 1 in, 1 out]
                        }
                      }
                      n229 = Index Array(array=w449, index=1) -> (element=→"DI 3":bool)
                      n230 = call "Conversion.vi"("Sensor Type"=w468, "Analog Channels"=w457) -> ("Converted Values"=w487:T7)  [unwired: 8 in, 1 out]
                      n231 = Index Array(array=w449, index=0) -> (element=→"DI 4":bool)
                      n232 = case shown="\"A1\", Default" "Sensor Selection" {
                        tunnel: w487 -> [w506 w513 w520 w527 w534 w541]
                        tunnel: [w505 w512 w519 w526 w533 w540] -> w462
                        tunnel: w469 -> [w501 w508 w515 w523 w529 w537]
                        tunnel: w468 -> [w504 w510 w517 w524 w531 w538]
                        tunnel: [w500 w507 w516 w522 w530 w536] -> w446
                        frame "A1", Default {
                          n233 = Unbundle(w504) -> ("Sensor 1"=w502:T3)  [unwired: 5 out]
                          n234 = To Unsigned Byte Integer(number=w502) -> (unsigned 8bit integer=w503:u8)
                          n235 = Unbundle(w506) -> ("Result"=w505:dbl)  [unwired: 5 out]
                          n236 = Index Array(array=w501, index=w503) -> (element=w500:cluster{string, string})
                        }
                        frame "A2" {
                          n237 = Unbundle(w510) -> ("Sensor 2"=w509:T3)  [unwired: 5 out]
                          n238 = To Unsigned Byte Integer(number=w509) -> (unsigned 8bit integer=w511:u8)
                          n239 = Unbundle(w513) -> ("Result"=w512:dbl)  [unwired: 5 out]
                          n240 = Index Array(array=w508, index=w511) -> (element=w507:cluster{string, string})
                        }
                        frame "A3" {
                          n241 = Unbundle(w517) -> ("Sensor 3"=w514:T3)  [unwired: 5 out]
                          n242 = To Unsigned Byte Integer(number=w514) -> (unsigned 8bit integer=w518:u8)
                          n243 = Unbundle(w520) -> ("Result"=w519:dbl)  [unwired: 5 out]
                          n244 = Index Array(array=w515, index=w518) -> (element=w516:cluster{string, string})
                        }
                        frame "A4" {
                          n245 = Unbundle(w524) -> ("Sensor 4"=w521:T3)  [unwired: 5 out]
                          n246 = To Unsigned Byte Integer(number=w521) -> (unsigned 8bit integer=w525:u8)
                          n247 = Unbundle(w527) -> ("Result"=w526:dbl)  [unwired: 5 out]
                          n248 = Index Array(array=w523, index=w525) -> (element=w522:cluster{string, string})
                        }
                        frame "A5" {
                          n249 = Unbundle(w531) -> ("Sensor 5"=w528:T3)  [unwired: 5 out]
                          n250 = Unbundle(w534) -> ("Result"=w533:dbl)  [unwired: 5 out]
                          n251 = To Unsigned Byte Integer(number=w528) -> (unsigned 8bit integer=w532:u8)
                          n252 = Index Array(array=w529, index=w532) -> (element=w530:cluster{string, string})
                        }
                        frame "A6" {
                          n253 = Unbundle(w538) -> ("Sensor 6"=w535:T3)  [unwired: 5 out]
                          n254 = To Unsigned Byte Integer(number=w535) -> (unsigned 8bit integer=w539:u8)
                          n255 = Unbundle(w541) -> ("Result"=w540:dbl)  [unwired: 5 out]
                          n256 = Index Array(array=w537, index=w539) -> (element=w536:cluster{string, string})
                        }
                      }
                      "Ylabel and Plot name" <- w446
                      n257 = Rotate 1D Array(1:w476, 2:1 ("n")) -> (0:w478:dbl[])
                      n258 = Rotate 1D Array(1:w473, 2:1 ("n")) -> (0:w474:dbl[])
                      n259 = Replace Array Subset(array=w478, new element=w462) -> (w438:dbl[])  [unwired: 1 in]
                      n260 = Replace Array Subset(array=w474, new element=w470) -> (w439:dbl[])  [unwired: 1 in]
                      n261 = Unbundle(w446) -> (w445:string)  [unwired: 1 out]
                      n262 = Build Array(w462) -> (w461:dbl[])
                      n263 = Build Array "Build Array"(w439, w438) -> (w440:dbl[][])
                      n264 = Reverse 1D Array(array=w439) -> (reversed array=w472:dbl[])
                      n265 = Reverse 1D Array(array=w438) -> (reversed array=w471:dbl[])
                      n266 = Transpose 2D Array(2D array=w440) -> (transposed array=w437:dbl[][])
                      n267 = Bundle(w472, w471) -> (→"XY Graph":cluster{dbl[], dbl[]})  [unwired: 1 in]
                      n268 = Number To Fractional String(number=w437, precision (6)=w443) -> (F-format string=→"ECG":string[][])  [unwired: 2 in]
                      n269 = TDMS Write(0:w465, 5:"bitalino", 7:w445, 9:w461, 11:w463) -> (4:w464:refnum<k34>, 15:w460:errorcluster)  [unwired: 1 in, 2 out]
                    }
                    frame Error {
                    }
                  }
                  "Consumer" <- w424
                }
                n270 = while {
                  tunnel: w378 -> [w403]
                  stop <- w400 stop-if-true
                  # "Update property nodes for every second"
                  n271 = Dequeue Element(queue=w403) -> (element=w401:bool, error out=w402:errorcluster)  [unwired: 2 in, 2 out]
                  n272 = case shown="No Error" w402 {
                    tunnel: w401 -> [w407 _]
                    tunnel: [FALSE TRUE] -> w400
                    frame No Error {
                      # "7."
                      n273 = property on="Ylabel and Plot name" class="Clust (strict)"() -> ("Value"=w410:cluster{string, string})  [unwired: 2 in, 2 out]
                      n274 = Unbundle(w410) -> (w409:string, w408:string)
                      n275 = property on="XY Graph" class="XYGraph (strict)"() -> ("YScale.NameLbl.Text"=w405:string)  [unwired: 2 in, 2 out]
                      n276 = property on="XY Graph" class="XYGraph (strict)"() -> ("Plot.Plot Name"=w404:string)  [unwired: 2 in, 2 out]
                      n277 = case shown="True" w407 {
                        tunnel: w405 -> [_ w416]
                        tunnel: w404 -> [_ w412]
                        tunnel: w409 -> [_ w413]
                        tunnel: w408 -> [_ w411]
                        frame False {
                        }
                        frame True {
                          n278 = Not Equal?(x=w416, y=w413) -> (x != y?=w414:bool)
                          n279 = Not Equal?(x=w412, y=w411) -> (x != y?=w415:bool)
                          n280 = case shown="True" w414 {
                            tunnel: w413 -> [_ w418]
                            frame False {
                            }
                            frame True {
                              n281 = property on="XY Graph" class="XYGraph (strict)"("YScale.NameLbl.Text"=w418) -> ()  [unwired: 2 in, 2 out]
                            }
                          }
                          n282 = case shown="True" w415 {
                            tunnel: w411 -> [_ w417]
                            frame False {
                            }
                            frame True {
                              n283 = property on="XY Graph" class="XYGraph (strict)"("Plot.Plot Name"=w417) -> ()  [unwired: 2 in, 2 out]
                            }
                          }
                        }
                      }
                    }
                    frame Error {
                    }
                  }
                }
                n284 = while {
                  shift-right: [w561] -> w390
                  shift-left: w396 -> [w551]
                  shift-right: [w562] -> w393
                  shift-left: w395 -> [w563]
                  shift-right: [w560] -> w392
                  shift-left: w361 -> [w550]
                  tunnel: w359 -> [w548]
                  i -> [w557]
                  stop <- w556 stop-if-true
                  # "Reading"
                  n285 = case shown="True" w548 {
                    tunnel: [w566 w575] -> w552
                    tunnel: w551 -> [w565 w569]
                    tunnel: w550 -> [w566 w568]
                    tunnel: [w565 w567] -> w549
                    frame False {
                    }
                    frame True {
                      # "5."
                      n286 = call "Digital IO.vi"("DO 4"="DO 4", "DO 3"="DO 3", "DO in"="DO 2", "DO 1"="DO 1") -> ("string"=w574:string)
                      n287 = VISA Write(VISA resource name=w568, write buffer=w574, error in (no error)=w569) -> (VISA resource name out=w575:refnum<visa-resource-name>, error out=w567:errorcluster)  [unwired: 1 out]
                    }
                  }
                  n288 = VISA Read(VISA resource name=w552, byte count=u32 8, error in (no error)=w549) -> (VISA resource name out=w560:refnum<visa-resource-name>, read buffer=w559:string, error out=w564:errorcluster)  [unwired: 1 out]
                  n289 = Enqueue Element(queue=w563, element=w559, error in (no error)=w564) -> (queue out=w562:refnum<queue>, error out=w561:errorcluster)  [unwired: 1 in, 1 out]
                  n290 = Unbundle By Name(w561) -> ("status"=w554:bool)
                  n291 = local read "Sync Stop"() -> (w555:bool)
                  n292 = local read "CRC Error"() -> (w553:bool)
                  n293 = Compound Arithmetic op=OR(w554, w555, w553) -> (w556:bool)
                  "producer" <- w557
                }
                n294 = call "Wait.vi"("error in (no error)"=w390) -> ("error out"=w391:errorcluster)  [unwired: 10 in]
                n295 = Build Array(u8 0) -> (w398:u8[])
                n296 = Byte Array To String(unsigned byte array=w398) -> (string=w397:string)
                n297 = VISA Write(VISA resource name=w392, write buffer=w397, error in (no error)=w391) -> (VISA resource name out=w388:refnum<visa-resource-name>, error out=w389:errorcluster)  [unwired: 1 out]
                n298 = VISA Close(VISA resource name=w388, error in (no error)=w389) -> (error out=w387:errorcluster)
                n299 = Release Queue(queue=w377, error in (no error)=w376) -> (error out=w363:errorcluster)  [unwired: 1 in, 2 out]
                n300 = Release Queue(queue=w393, error in (no error)=w387) -> (error out=w385:errorcluster)  [unwired: 1 in, 2 out]
                n301 = TDMS Close(8:w363, 11:w362) -> ()  [unwired: 2 out]
                n302 = Generate User Event(user event=w386, event data cluster=w385) -> ()  [unwired: 2 in, 2 out]
              }
              frame Error {
                n303 = Generate User Event(user event=w577, event data cluster=w576) -> ()  [unwired: 2 in, 2 out]
              }
            }
          }
          frame "Exit" {
            n304 = flat-sequence {
              frame #0 {
                n305 = property on="Stop Button" class="Bool"("DisabledEnum"=T4."Enabled" ("Disabled")) -> ()  [unwired: 2 in, 2 out]
              }
              frame #1 {
                n306 = Stop(stop? (T)=TRUE) -> ()
              }
            }
          }
        }
        "Status" <- w253
      }
      frame Error {
      }
    }
  }
  n307 = Release Queue(queue=w21, error in (no error)=w20) -> (error out=w8:errorcluster)  [unwired: 1 in, 2 out]
  n308 = Unregister For Events(event registration refnum=w7, error in=w8) -> (error out=w6:errorcluster)
  n309 = Destroy User Event(user event=w5, error in=w6) -> ()  [unwired: 1 out]
